vi "Load_Source.vi"(8 "error in (no error)":errorcluster, 11 "AB_Build in":refnum<class "AB_Build.lvclass">) -> (0 "error out":errorcluster, 3 "AB_Build out":refnum<class "AB_Build.lvclass">)   [LabVIEW 2020, in "AB_Build.lvclass"]
uses:
  <vilib>/AppBuilder/AB_Classes/Build/AB_Build.lvclass
  <vilib>/AppBuilder/AB_Classes/Build/AB_Build.lvclass/AB_Build.ctl
  <vilib>/AppBuilder/AB_Classes/Source/AB_Source.lvclass
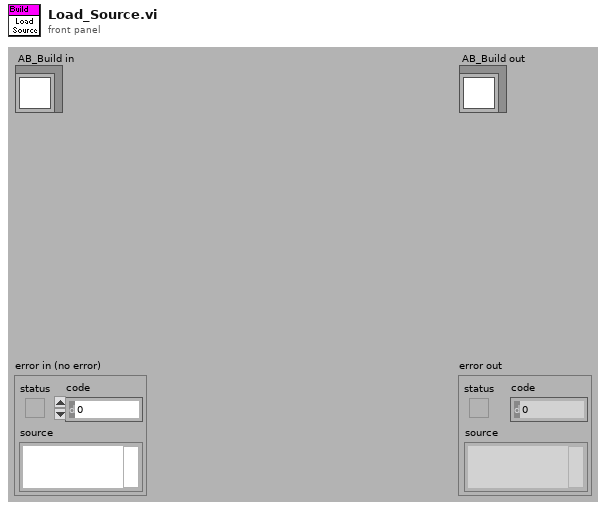
[diagram p1: front panel]
types:
  T1 = typedef "ItemRef.ctl" = u64
  T2 = typedef "AB_Source.ctl" = cluster{"path":path, "itemID":string, "parentIndex":i32, "sourceInclusion":T3, "destinationIndex":i32, "properties":T4[], "newName":string, "lvfile":bool, "valid":bool, "eng_inBuild":bool, "eng_isNonVILink":bool, "Amalgamation":bool, "Amalgamation Piece":bool, "eng_delimitedName":string, "preventRename":bool}
  T3 = typedef "AB_Source_Inclusion.ctl" = enum16{"IncludeIfReferenced", "Include", "Exclude", "TopLevel"}
  T4 = typedef "AB_Source_Properties.ctl" = cluster{"sourcePropertyType":T5, "value":variant}
  T5 = typedef "AB_Source_Property_Type.ctl" = enum16{"Remove block diagram", "Remove front panel", "Password", "Window has title bar", "Show menu bar", "Show vertical scroll bar", "Show horizontal scroll bar", "Show toolbar", "Show Abort button", "Show fp when called", "Window behavior", "Allow user to close window", "Window run-time position", "Run when opened", "Allow debugging", "Auto error handling", "Generate guard code", "Use stack variables", "Expression folding", "Integer only", "Inline subVI"}
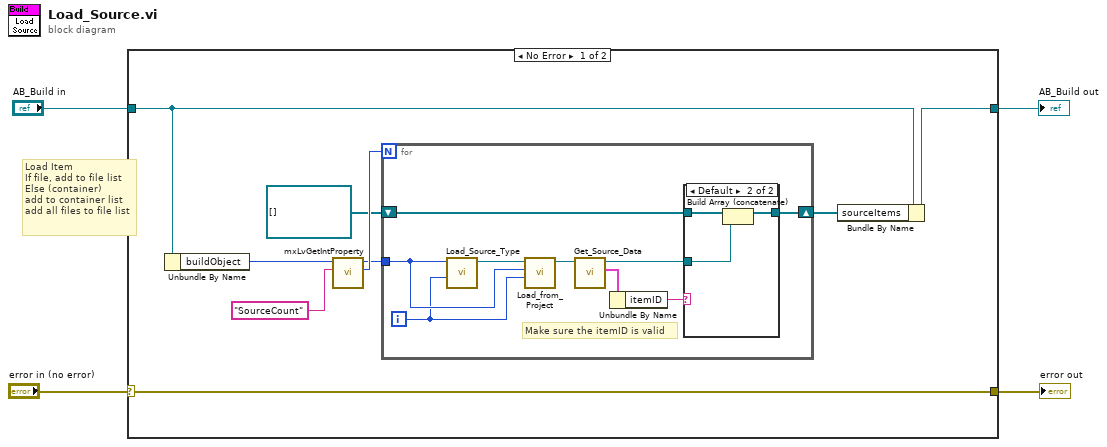
[diagram p0: block diagram]
diagram:
  # "Load Item\nIf file, add to file list\nElse (container)\nadd to container list\nadd all files to file list"
  n1 = case shown="No Error" "error in (no error)" {
    selector: "error in (no error)" -> [w13 w28]
    tunnel: [w13 w28] -> w3
    tunnel: [w10 w27] -> w1
    tunnel: "AB_Build in" -> [w9 w27]
    frame No Error {
      n2 = Unbundle By Name(w9) -> ("buildObject"=w8:T1)
      n3 = call <resource>:"mxLvGetIntProperty.vi"("Tag"="SourceCount", "Item"=w8) -> ("Value"=w12:i32, "Item"=w11:T1)  [unwired: 7 in, 1 out]
      n4 = for {
        N: w12 -> [_]
        tunnel: w11 -> [w22]
        shift-right: [w17] -> w5
        shift-left: refnum<class "AB_Source.lvclass">[] [] -> [w16]
        i -> [w20]
        # "Make sure the itemID is valid"
        n5 = call <vilib>:"Load_Source_Type.vi"("index"=w20, "buildObject"=w22) -> ("AB_Source out"=w21:refnum<class "AB_Source.lvclass">)  [unwired: 8 in, 1 out]
        n6 = call-dynamic "Load_from_Project.vi"("index"=w20, "buildObject"=w22, "AB_Source in"=w21) -> ("AB_Source out"=w19:refnum<class "AB_Source.lvclass">)  [unwired: 6 in, 2 out]
        n7 = call <vilib>:"Get_Source_Data.vi"("Class in"=w19) -> ("data"=w15:T2, "Class out"=w18:refnum<class "AB_Source.lvclass">)  [unwired: 8 in, 1 out]
        n8 = Unbundle By Name(w15) -> ("itemID"=w14:string)
        n9 = case shown="Default" w14 {
          tunnel: w18 -> [_ w26]
          tunnel: [w23 w25] -> w17
          tunnel: w16 -> [w23 w24]
          frame "" {
          }
          frame Default {
            n10 = Build Array (concatenate)(w24, w26) -> (w25:refnum<class "AB_Source.lvclass">[])
          }
        }
      }
      n11 = Bundle By Name(cluster=w9, "sourceItems"=w5) -> (w10:refnum<class "AB_Build.lvclass">)
    }
    frame Error {
    }
  }
  "error out" <- w3
  "AB_Build out" <- w1
